vi "DSF.Engine.Memory.Pointer.VS Channels.New.vi"(8 "error in (no error)":errorcluster, 10 "channel count":u64, 11 "Data Reference":T1 format="%.0x") -> (0 "error out":errorcluster, 3 "VS Channels Pointer out":refnum<class "DSF.Engine.Memory.Pointer.VS Channels.lvclass">)   [LabVIEW 2016, in "DSF.Engine.lvlib" / "DSF.Engine.Memory.Pointer.VS Channels.lvclass"]
uses:
  DSF.Engine.Memory.Pointer.VS Channels.lvclass
  C:/Git/SourceTree/DSF/Source/Submodules/Memory/Source/Classes/External/Memory.Pointer.External.lvclass
  <vilib>/NI Veristand/Custom Device API/Data Reference.ctl
  Shared/Typedefs/DSF.Shared.Typedefs.Data Type.ctl
  Shared/VIs/DSF.Shared.Data Type.Sizeof.vi
  <vilib>/NI Veristand/Custom Device API/Global Data Refs.vi
  DSF.Shared.lvlib
  Submodules/Memory/Source/Classes/External/Memory.Pointer.External.lvclass
  <vilib>/NI Veristand/Custom Device API/Custom Device API.lvlib
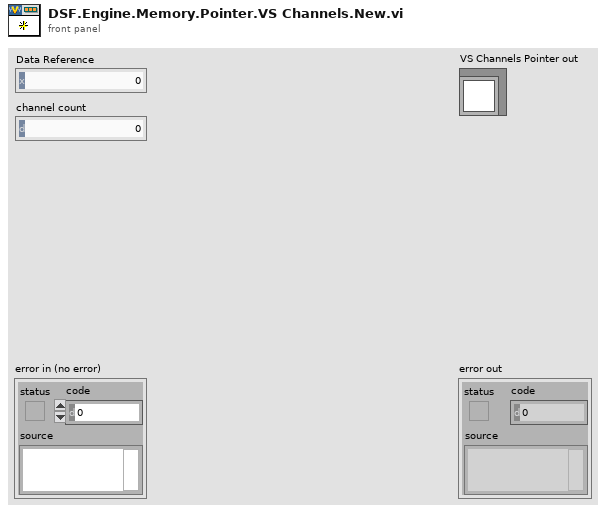
[diagram p1: front panel]
types:
  T1 = typedef "Custom Device API.lvlib/Data Reference.ctl" = i32
  T2 = typedef "DSF.Shared.lvlib/DSF.Shared.Typedefs.Data Type.ctl" = enum8{"Bool", "SGL", "DBL", "I8", "I16", "I32", "I64", "U8", "U16", "U32", "U64"}
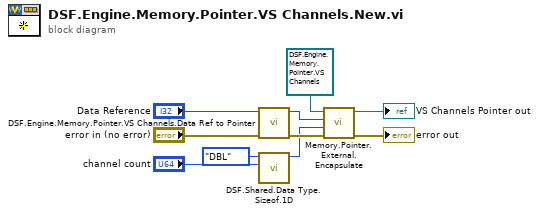
[diagram p0: block diagram]
diagram:
  n1 = call "DSF.Engine.Memory.Pointer.VS Channels.Data Ref to Pointer.vi"("error in (no error)"="error in (no error)", "Data Reference"="Data Reference") -> ("error out"=w6:errorcluster, "Channel Pointer"=w4:u64)  [unwired: 8 in]
  n2 = call "DSF.Shared.Data Type.Sizeof.1D.vi"("count"="channel count", "data type"=DSF.Shared.Typedefs.Data_Type."DBL") -> ("size in bytes"=w3:u64)  [unwired: 9 in]
  n3 = call "Memory.Pointer.External.Encapsulate.vi"("error in (no error)"=w6, "size"=w3, "address"=w4, "external pointer in"=refnum<class "DSF.Engine.Memory.Pointer.VS Channels.lvclass"> refnum ("VS Channels Pointer out")) -> ("error out"=→"error out":errorcluster, "external pointer out"=→"VS Channels Pointer out":refnum<class "DSF.Engine.Memory.Pointer.VS Channels.lvclass">)  [unwired: 6 in]
